vi "Write Simple smFRET Photon-HDF5 File.vi"(7 "Metadata":T1={"Setup (Mandatory)"={"num_pixels"=2, "num_spots"=1, "num_spectral_ch"=2, "num_polarization_ch"=1, "num_split_ch"=1, "modulated_excitation"=FALSE, "lifetime"=FALSE}, "Excitation Types"=[FALSE], "detection_wavelengths"=[5.800000000000001e-07, 6.4e-07], "excitation_wavelengths"=[5.32e-07], "Photon Data"={"Time Stamp Unit"=1e-08, "Measurement Type"=enum."smFRET", "Spectral Channels List"=[{"Detector IDs"=[0]}, {"Detector IDs"=[1]}]}, "Description"="this is a description", "Sample"={"sample_name"="Sample Name", "buffer_name"="Buffer Name", "dye_names"="Cy3B, ATTO647N"}, "Identity"={"author"="Author Name", "author_affiliation"="Company Name"}, "Provenance"={"filename"="File Name", "software"="Acquisition Software"}}, 8 "Error In":errorcluster, 9 "Photon Time Stamps":i64[](array[numeric]), 10 "Photon Detector IDs":u8[](array[numeric]), 11 "File Path Control":path) -> (0 "Error Out":errorcluster)   [LabVIEW 2010]
panel:
  # "Photon Data"
  # "Setup (Optional)"
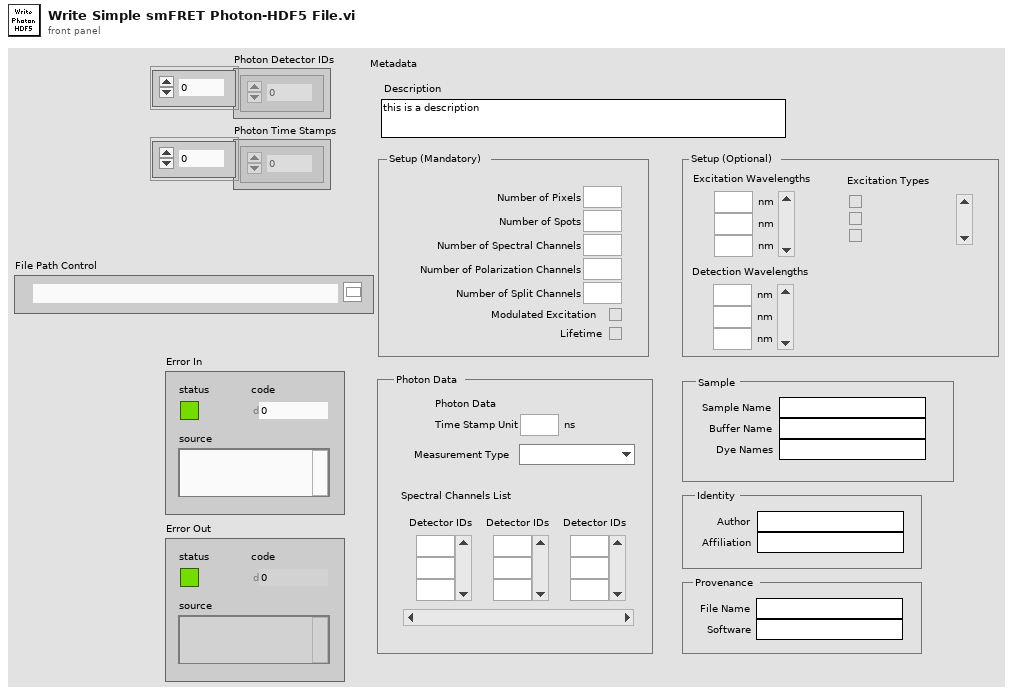
[diagram p1: front panel]
types:
  T1 = cluster{"Setup (Mandatory)":cluster{"num_pixels":u8, "num_spots":u8, "num_spectral_ch":u8, "num_polarization_ch":u8, "num_split_ch":u8, "modulated_excitation":bool, "lifetime":bool}, "Excitation Types":bool[], "detection_wavelengths":dbl[unit][], "excitation_wavelengths":dbl[unit][], "Photon Data":cluster{"Time Stamp Unit":dbl[unit], "Measurement Type":enum16{"Undefined", "smFRET"}, "Spectral Channels List":cluster{"Detector IDs":u8[]}[]}, "Description":string, "Sample":cluster{"sample_name":string, "buffer_name":string, "dye_names":string}, "Identity":cluster{"author":string, "author_affiliation":string}, "Provenance":cluster{"filename":string, "software":string}}
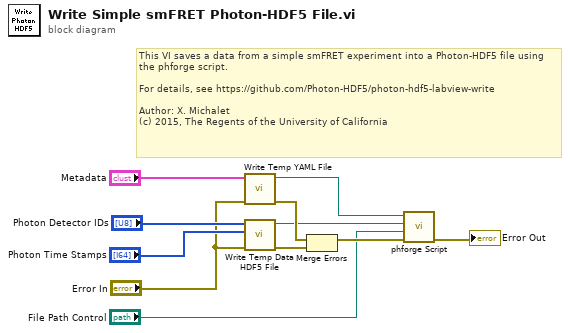
[diagram p0: block diagram]
diagram:
  # "This VI saves a data from a simple smFRET experiment into a Photon-HDF5 file using the phforge script.\n\nFor details, see https://github.com/Photon-HDF5/photon-hdf5-labview-write\n\nAuthor: X. Michalet\n(c) 2015, The Regents of the University of California"
  n1 = call "Write Temp YAML File.vi"("Error In"="Error In", "Metadata"="Metadata") -> ("Error Out"=w7:errorcluster, "Temp YAML File"=w4:path)  [unwired: 8 in]
  n2 = call "Write Temp Data HDF5 File.vi"("Error In"="Error In", "Photon Time Stamps"="Photon Time Stamps", "Photon Detector IDs"="Photon Detector IDs") -> ("Error Out"=w6:errorcluster, "HDF5 File Path"=w3:path)  [unwired: 7 in]
  n3 = Merge Errors(w7, w6) -> (w5:errorcluster)
  n4 = call "phforge Script.vi"("Error in"=w5, "Output File Path"="File Path Control", "HDF5 File Path"=w3, "Metadata File Path"=w4) -> ("Error out"=→"Error Out":errorcluster)  [unwired: 4 in, 3 out]
